vi "Configure Channel (Threshold Voltage).vi"(7 "Event Type (1: Start)":i32(ring)=1 items=["Start"=1, "Stop"=2], 8 "error in (no error)":errorcluster, 9 "Threshold Voltage (0 V)":dbl, 10 "Channel (1: Channel 1)":i32(ring)=1 items=["Channel 1"=1, "Channel 2"=2], 11 "VISA resource name":refnum<visa-resource-name>) -> (0 "error out":errorcluster, 3 "VISA resource name out":refnum<visa-resource-name>)   [LabVIEW 2024, in "Agilent 532XX Series.lvlib"]
doc: "Configures the threshold voltage characteristics of input channel with the auto-leveling disabled."
uses:
  Agilent 532XX Series.lvlib
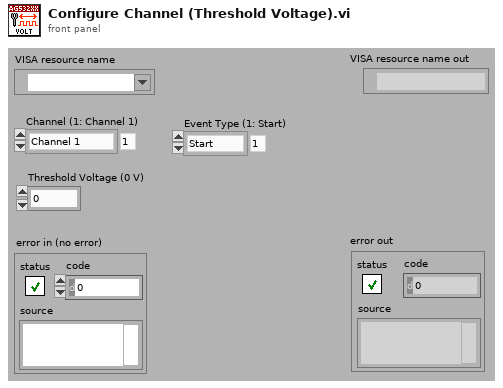
[diagram p1: front panel]
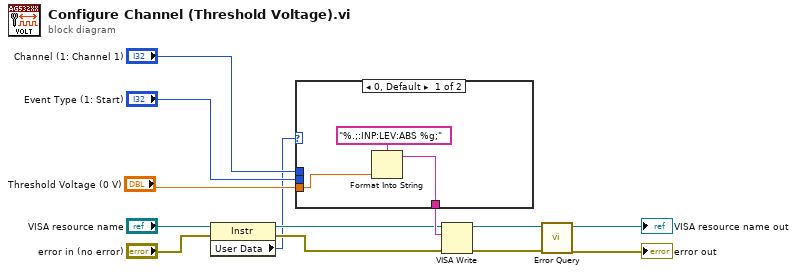
[diagram p0: block diagram]
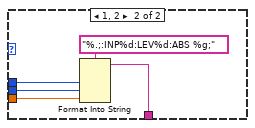
[diagram p2: hidden frame]
diagram:
  n1 = property class="Instr"(reference="VISA resource name", error in="error in (no error)") -> (reference out=w4:refnum<visa-resource-name>, error out=w2:errorcluster, "User Data"=w1:u32)
  n2 = case shown="0, Default" w1 {
    tunnel: "Channel (1: Channel 1)" -> [_ w20]
    tunnel: "Event Type (1: Start)" -> [_ w19]
    tunnel: [w14 w18] -> w11
    tunnel: "Threshold Voltage (0 V)" -> [w15 w17]
    frame 0, Default {
      n3 = Format Into String(format string="%.;:INP:LEV:ABS %g;", w15) -> (resulting string=w14:string)  [unwired: 2 in, 1 out]
    }
    frame 1, 2 {
      n4 = Format Into String(format string="%.;:INP%d:LEV%d:ABS %g;", w20, w19, w17) -> (resulting string=w18:string)  [unwired: 2 in, 1 out]
    }
  }
  n5 = VISA Write(VISA resource name=w4, write buffer=w11, error in (no error)=w2) -> (VISA resource name out=w10:refnum<visa-resource-name>, error out=w9:errorcluster)  [unwired: 1 out]
  n6 = call "Error Query.vi"("error in (no error)"=w9, "VISA resource name"=w10) -> ("error out"=→"error out":errorcluster, "VISA resource name out"=→"VISA resource name out":refnum<visa-resource-name>)  [unwired: 8 out]
